vi "QuerySystemDefinitionFile.vi"(8 "error in (no error)":errorcluster, 11 "System Definiton File in":path) -> (0 "error out":errorcluster, 3 "System Definition Information out":T1)   [LabVIEW 2027, in "VeriStandTestUtilities.lvlib"]
uses:
  VeriStandTestUtilities.lvlib
  SystemDefinitionInformation.ctl
  TargetInformation.ctl
  ChassisInformation.ctl
panel:
  in  "System Definition Information":T1
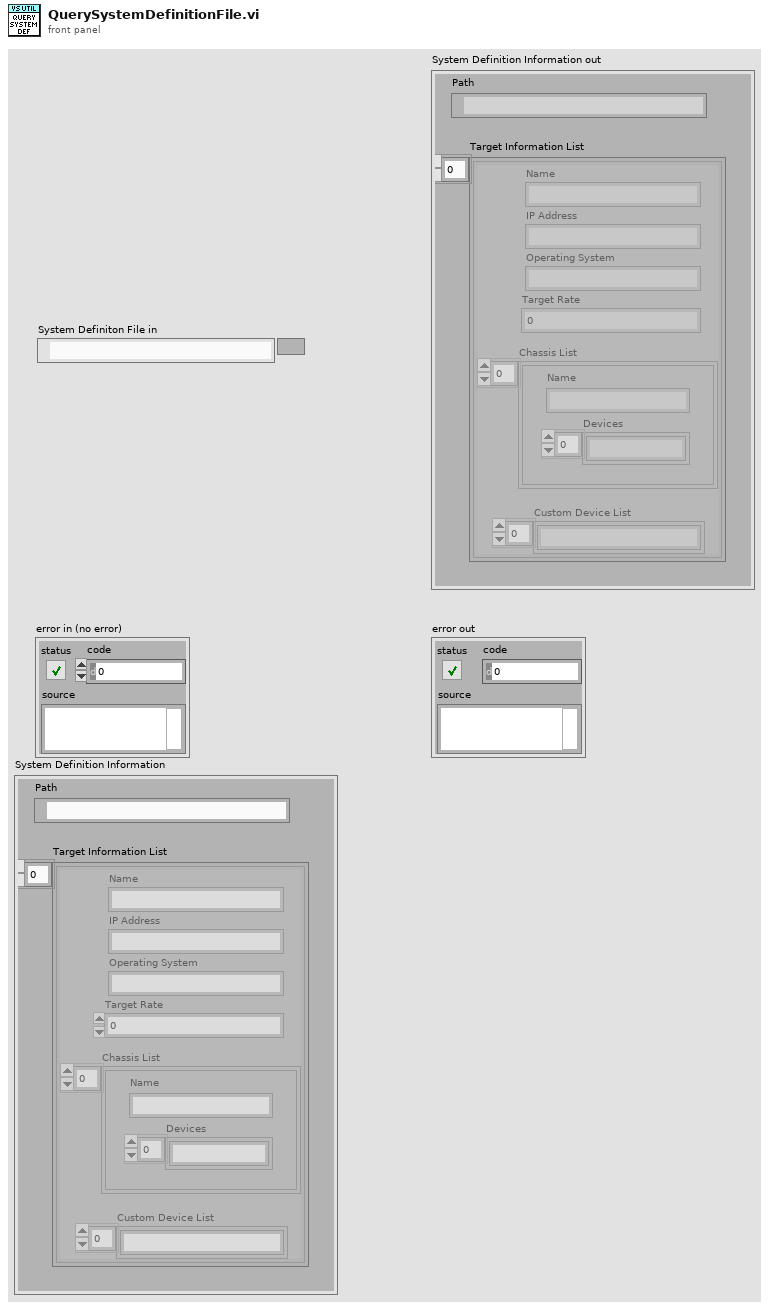
[diagram p1: front panel]
types:
  T1 = typedef "VeriStandTestUtilities.lvlib/SystemDefinitionInformation.ctl" = cluster{"Path":path, "Target Information List":T2[]}
  T2 = typedef "VeriStandTestUtilities.lvlib/TargetInformation.ctl" = cluster{"Name":string, "IP Address":string, "Operating System":string, "Target Rate":dbl, "Chassis List":T3[], "Custom Device List":string[]}
  T3 = typedef "VeriStandTestUtilities.lvlib/ChassisInformation.ctl" = cluster{"Name":string, "Devices":string[]}
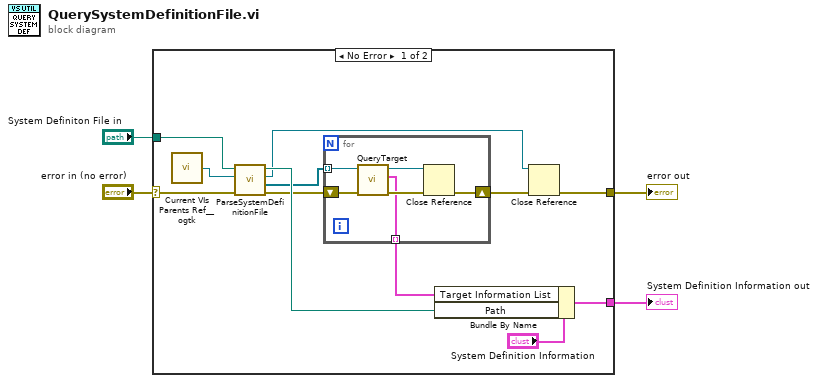
[diagram p0: block diagram]
diagram:
  n1 = case shown="No Error" "error in (no error)" {
    selector: "error in (no error)" -> [w12 w23]
    tunnel: [w6 w23] -> w3
    tunnel: "System Definiton File in" -> [w11 _]
    tunnel: [w14 _] -> w1
    frame No Error {
      n2 = call <userlib>:"Current VIs Parents Ref__ogtk.vi"() -> ("Calling VI's Reference"=w10:refnum<vi>)  [unwired: 2 in]
      n3 = call "ParseSystemDefinitionFile.vi"("error in (no error)"=w12, "VI in"=w10, "System Definiton File in"=w11) -> ("error out"=w8:errorcluster, "Target List out"=w7:refnum<k39>[], "NationalInstruments.VeriStand.SystemDefinitionAPI.SystemDefinition"=w5:refnum<k39>, "Absolute System Definiton File out"=w9:path)  [unwired: 5 in]
      n4 = for {
        shift-right: [w20] -> w13
        shift-left: w8 -> [w22]
        tunnel: [w18] -> w15 mode=indexing
        tunnel: w7 -> [w17] mode=indexing
        n5 = call "QueryTarget.vi"("error in (no error)"=w22, "NationalInstruments.VeriStand.SystemDefinitionAPI.Target"=w17) -> ("error out"=w21:errorcluster, "Target Information"=w18:T2, "NationalInstruments.VeriStand.SystemDefinitionAPI.Target"=w19:refnum<k39>)  [unwired: 7 in]
        n6 = Close Reference(reference=w19, error in (no error)=w21) -> (error out=w20:errorcluster)
      }
      n7 = Bundle By Name(cluster="System Definition Information", "Target Information List"=w15, "Path"=w9) -> (w14:T1)
      n8 = Close Reference(reference=w5, error in (no error)=w13) -> (error out=w6:errorcluster)
    }
    frame Error {
    }
  }
  "error out" <- w3
  "System Definition Information out" <- w1
